vi "Query ViBoolean.vi"(8 "error in (no error)":errorcluster, 9 "Query":string, 11 "VISA resource name":refnum<visa-resource-name>) -> (0 "error out":errorcluster, 2 "Response Value":bool, 3 "VISA resource name out":refnum<visa-resource-name>)   [LabVIEW 2020, in "Rohde&Schwarz CMWXP NR FR1 Measurement.lvlib"]
doc: "This VI sends the SCPI query to the instrument, reads the response and converts it to boolean value."
uses:
  <instrlib>/Rohde&Schwarz CMWXP NR FR1 Measurement/Rohde&Schwarz CMWXP NR FR1 Measurement.lvlib
  <instrlib>/Rohde&Schwarz CMWXP NR FR1 Measurement/Private/rsidr_core.llb/rsidr_core.lvlib
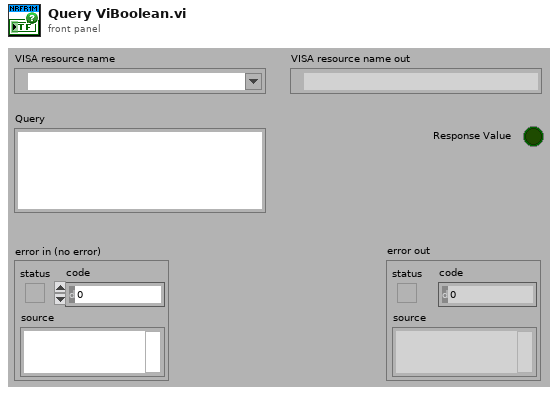
[diagram p1: front panel]
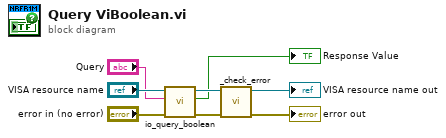
[diagram p0: block diagram]
diagram:
  n1 = call <instrlib>:"io_query_boolean.vi"("error in"="error in (no error)", "write buffer"="Query", "VISA resource name"="VISA resource name") -> ("error out"=w6:errorcluster, "boolean value out"=→"Response Value":bool, "VISA resource name out"=w5:refnum<visa-resource-name>)  [unwired: 6 in]
  n2 = call <instrlib>:"_check_error.vi"("error in (no error)"=w6, "VISA resource name"=w5) -> ("error out"=→"error out":errorcluster, "VISA resource name out"=→"VISA resource name out":refnum<visa-resource-name>)  [unwired: 8 in]
